vi "Acquired points counter exit logic.vi"(9 "Initial reset":bool, 10 "Number of samples to be acquired in each trial (i.e. Target samples)":u64, 11 "Running Count (current trial)":u64) -> (1 "Reset fail-safe timeout":bool, 3 "Stop acquisition loop":bool)   [LabVIEW 2017]
panel:
  out "Target -1 reached and \nno further points returned":bool
  out "Target reached":bool
  # "RE-ENTRANT"
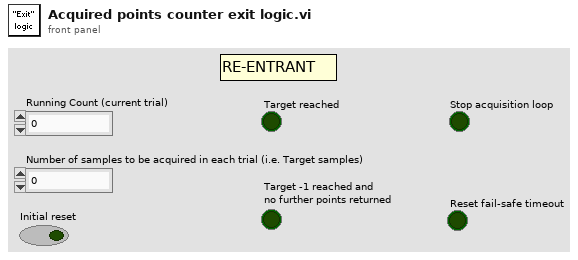
[diagram p1: front panel]
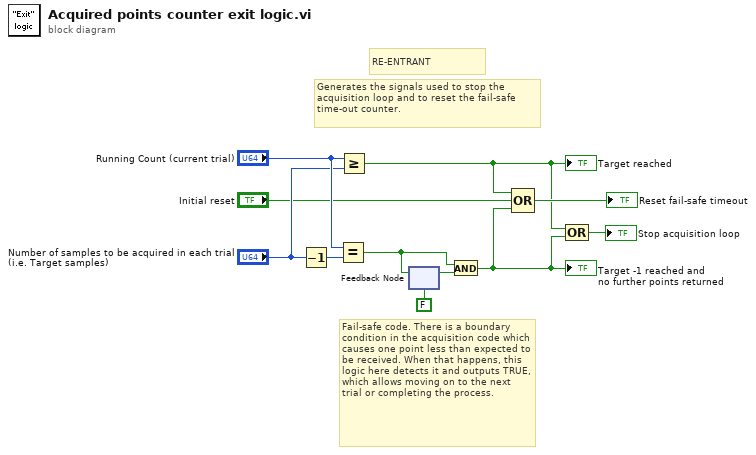
[diagram p0: block diagram]
diagram:
  # "Fail-safe code. There is a boundary condition in the acquisition code which causes one point less than expected to be received. When that happens, this logic here detects it and outputs TRUE, which allows moving on to the next trial or completing the process."
  # "Generates the signals used to stop the acquisition loop and to reset the fail-safe time-out counter."
  # "RE-ENTRANT"
  n1 = Decrement(x="Number of samples to be acquired in each trial (i.e. Target samples)") -> (x-1=w5:u64)
  n2 = Equal?(x="Running Count (current trial)", y=w5) -> (x = y?=w7:bool)
  n3 = Greater Or Equal?(x="Running Count (current trial)", y="Number of samples to be acquired in each trial (i.e. Target samples)") -> (x >= y?=w3:bool)
  "Target reached" <- w3
  n4 = feedback #1(FALSE) -> (w6:bool)
  n5 = feedback-in #1(w7) -> ()
  n6 = And(x=w7, y=w6) -> (x .and. y?=w2:bool)
  "Target -1 reached and \nno further points returned" <- w2
  n7 = Compound Arithmetic op=OR(w3, "Initial reset", w2) -> (→"Reset fail-safe timeout":bool)
  n8 = Compound Arithmetic op=OR(w3, w2) -> (→"Stop acquisition loop":bool)
